vi "main.vi"() -> ()   [LabVIEW 2015]
panel:
  in  "Command":string
  in  "불리언":bool
  out "Resoponse":string
  in  "Delay Time":u32
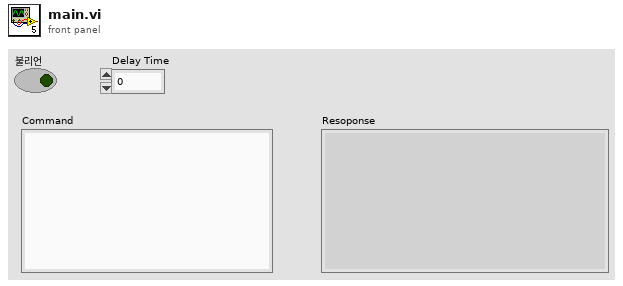
[diagram p1: front panel]
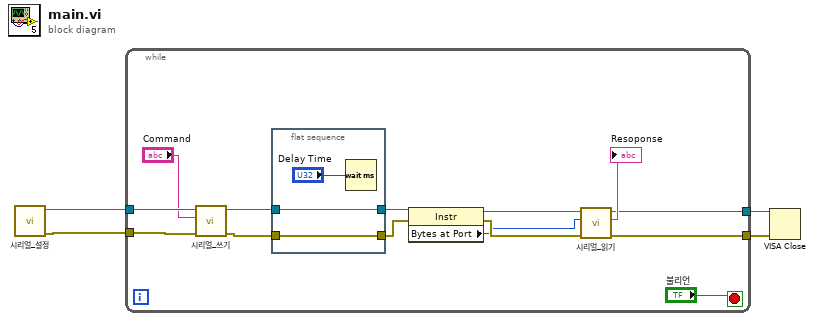
[diagram p0: block diagram]
diagram:
  n1 = call "시리얼_설정.vi"() -> ("Error Out"=w3:errorcluster, "VISA resource name out"=w4:refnum<visa-resource-name>)  [unwired: 10 in]
  n2 = while {
    tunnel: w4 -> [w18]
    tunnel: w3 -> [w17]
    tunnel: [w7] -> w2
    tunnel: [w6] -> w1
    stop <- "불리언" stop-if-true
    n3 = call "시리얼_쓰기.vi"("Error In"=w17, "Command"="Command", "VISA 리소스 이름"=w18) -> ("Error Out"=w15:errorcluster, "VISA 리소스 이름 출력"=w16:refnum<visa-resource-name>)  [unwired: 7 in]
    n4 = flat-sequence {
      tunnel: w16 -> [w20]
      tunnel: [w20] -> w12
      tunnel: w15 -> [w19]
      tunnel: [w19] -> w11
      frame #0 {
        n5 = Wait (ms)(milliseconds to wait="Delay Time") -> ()  [unwired: 1 out]
      }
    }
    n6 = property class="Instr"(reference=w12, error in=w11) -> (reference out=w10:refnum<visa-resource-name>, error out=w9:errorcluster, "Bytes at Port"=w8:u32)
    n7 = call "시리얼_읽기.vi"("Error In"=w9, "바이트 카운트"=w8, "VISA 리소스 이름"=w10) -> ("Error Out"=w6:errorcluster, "Resoponse"=→"Resoponse":string, "VISA 리소스 이름 출력"=w7:refnum<visa-resource-name>)  [unwired: 5 in, 1 out]
  }
  n8 = VISA Close(VISA resource name=w2, error in (no error)=w1) -> ()  [unwired: 1 out]
